vi "To XML - With Package - Returns XML Entities.vi"() -> ()   [LabVIEW 2017, in "Cobertura.Tests.lvlib" / "Coverage.lvlib"]
uses:
  Coverage.lvlib
  <vilib>/xml/Close Reference(Node).vi
  Cobertura/Coverage/Coverage.lvclass
  <vilib>/xml/NI_XML.lvlib
  <resource>/objmgr/DOMUserDefRef.rc
  <vilib>/PNR/Transparent Assertions/Transparent Assertions/Transparent Assertions.lvlib
  Cobertura/Package/Package.lvclass
panel:
  out "error out":errorcluster
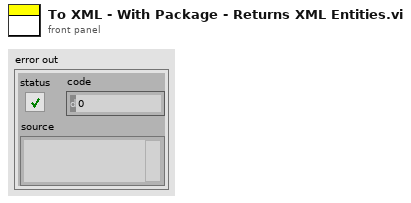
[diagram p1: front panel]
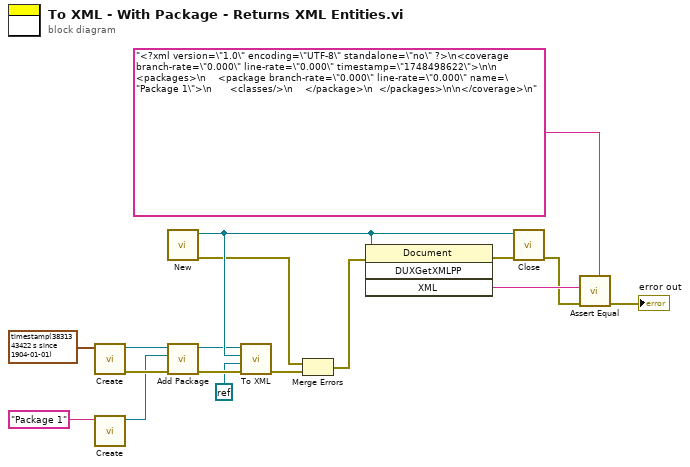
[diagram p0: block diagram]
diagram:
  n1 = call "Create.vi"("Timestamp"=timestamp(3831343422.3303647 s since 1904-01-01)) -> ("error out"=w17:errorcluster, "Coverage"=w5:refnum<class "Coverage.lvclass">)  [unwired: 9 in]
  n2 = call "Create.vi"("Name"="Package 1") -> ("Package"=w4:refnum<class "Package.lvclass">)  [unwired: 9 in, 1 out]
  n3 = call <vilib>:"New.vi"() -> ("error out"=w3:errorcluster, "DOM document out"=w15:refnum<k20>)  [unwired: 8 in]
  n4 = call "Add Package.vi"("error in (no error)"=w17, "Package"=w4, "Coverage in"=w5) -> ("error out"=w9:errorcluster, "Coverage out"=w8:refnum<class "Coverage.lvclass">)  [unwired: 7 in]
  n5 = call-dynamic "To XML.vi"("error in (no error)"=w9, "Parent"=refnum<k0> refnum, "Document"=w15, "Coverage in"=w8) -> ("error out"=w10:errorcluster)  [unwired: 7 in]
  n6 = Merge Errors(w3, w10) -> (w11:errorcluster)
  n7 = invoke class="Document" method="DUXGetXMLPP"(reference=w15, error in=w11) -> (error out=w16:errorcluster, "XML"=w14:string)  [unwired: 2 in, 2 out]
  n8 = call-poly <vilib>:"Close.vi"("error in (no error)"=w16, "node"=w15) -> ("error out"=w2:errorcluster)  [unwired: 7 in]
  n9 = call <vilib>:"Assert Equal.vi"("Expected"="<?xml version=\"1.0\" encoding=\"UTF-8\" standalone=\"no\" ?>\n<coverage branch-rate=\"0.000\" line-rate=\"0.000\" timestamp=\"1748498622\">\n\n  <packages>\n    <package branch-rate=\"0.000\" line-rate=\"0.000\" name=\"Package 1\">\n      <classes/>\n    </package>\n  </packages>\n\n</coverage>\n", "error in (no error)"=w2, "Actual"=w14) -> ("error out"=→"error out":errorcluster)  [unwired: 8 in]
